vi "sub vi - Initialize Video.vi"   [LabVIEW 2010]
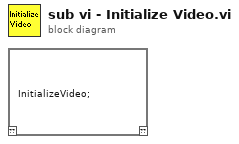
[diagram p0: block diagram]
diagram:
  n1 = script code="InitializeVideo;"() -> ()  [unwired: 2 out]
